vi "LVPresent_Globals.vi"() -> ()   [LabVIEW 2012]
uses:
  <vilib>/Utility/miscctls.llb/LVBoundsTypeDef.ctl
  <vilib>/Utility/miscctls.llb/LVPositionTypeDef.ctl
panel:
  in  "multiplier":sgl=1.1
  in  "offset":sgl=0.1
  in  "panel offset":T1={"Left"=-41, "Top"=-34}
  in  "Resolution":i32=10
  in  "EndSlide":bool
  in  "Scene Refnum":refnum<vi>
  in  "Side Bounds":T2
  # "Thumbs"
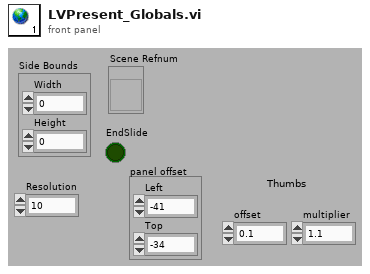
[diagram p1: front panel]
types:
  T1 = typedef "LVPositionTypeDef.ctl" = cluster{"Left":i32, "Top":i32}
  T2 = typedef "LVBoundsTypeDef.ctl" = cluster{"Width":u32, "Height":u32}
diagram:
